vi "Parse Channel Strings.vi"(1 "Channels Info":T1[](array[typedef])) -> (0 "Channel Strings":string[](array[string]))   [LabVIEW 2021, in "myRIO Channel List.xctl"]
uses:
  <vilib>/myRIO/Common/Express VI Framework/xctls/myRIO Channel List/myRIO Channel List.xctl
  <vilib>/myRIO/Common/Profile Manager Framework/typedefs/Channel Info.ctl
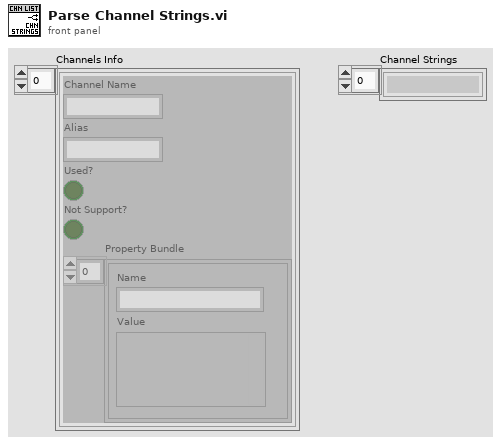
[diagram p1: front panel]
types:
  T1 = typedef "Channel Info.ctl" = cluster{"Channel Name":string, "Alias":string, "Used?":bool, "Not Support?":bool, "Property Bundle":cluster{"Name":string, "Value":variant}[]}
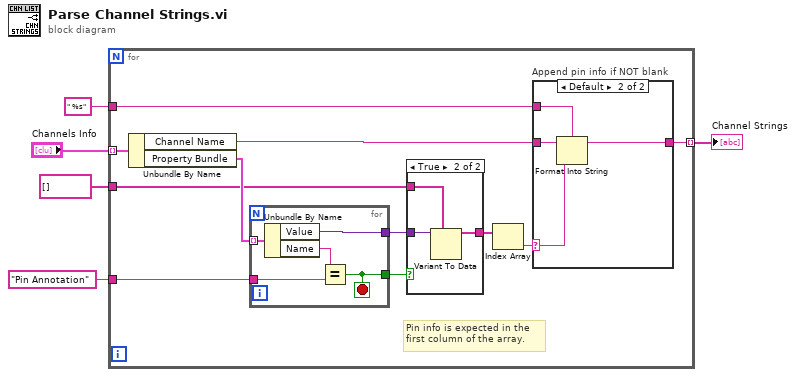
[diagram p0: block diagram]
diagram:
  n1 = for {
    tunnel: "Channels Info" -> [w15] mode=indexing
    tunnel: [w16] -> w1 mode=indexing
    tunnel: "Pin Annotation" ("Name") -> [w8]
    tunnel: string[] [] -> [w7]
    tunnel: " %s" ("format string") -> [w6]
    # "Pin info is expected in the first column of the array."
    n2 = Unbundle By Name(w15) -> ("Channel Name"=w14:string, "Property Bundle"=w9:cluster{"Name":string, "Value":variant}[])
    n3 = for {
      tunnel: w9 -> [w21] mode=indexing
      tunnel: w8 -> [w19]
      tunnel: [w18] -> w13
      tunnel: [w17] -> w12
      stop <- w17 stop-if-true
      n4 = Unbundle By Name(w21) -> ("Value"=w18:variant, "Name"=w20:string)
      n5 = Equal?(x=w20, y=w19) -> (x = y?=w17:bool)
    }
    n6 = case shown="True" w12 {
      tunnel: w13 -> [_ w25]
      tunnel: [w22 w24] -> w11
      tunnel: w7 -> [w22 w23]
      frame False {
      }
      frame True {
        n7 = Variant To Data(type=w23, Variant=w25) -> (data=w24:string[])  [unwired: 1 in, 1 out]
      }
    }
    n8 = Index Array(array=w11) -> (element=w10:string)  [unwired: 1 in]
    n9 = case "Append pin info if NOT blank" shown="Default" w10 {
      selector: w10 -> [_ w27]
      tunnel: w14 -> [w26 w30]
      tunnel: [w26 w29] -> w16
      tunnel: w6 -> [_ w28]
      frame "" {
      }
      frame Default {
        n10 = Format Into String(format string=w28, initial string=w30, w27) -> (resulting string=w29:string)  [unwired: 1 in, 1 out]
      }
    }
  }
  "Channel Strings" <- w1
